vi "Write Operator.vi"(7 "Send any changes now? (F)":bool, 8 "error in (no error)":errorcluster, 10 "Operator":string caption="DUT Serial", 11 "Fiber Auto Collimation state data in":refnum<class "Fiber Auto Collimation state data.lvclass">) -> (0 "error out":errorcluster, 3 "Fiber Auto Collimation state data out":refnum<class "Fiber Auto Collimation state data.lvclass">)   [LabVIEW 2018, in "Fiber Auto Collimation state data.lvclass"]
doc: "Serial number of the Device Under Test on the station at the moment."
uses:
  Fiber Auto Collimation state data.lvclass
  Fiber Auto Collimation state data.lvclass/Fiber Auto Collimation state data.ctl
  Tracked state data.ctl
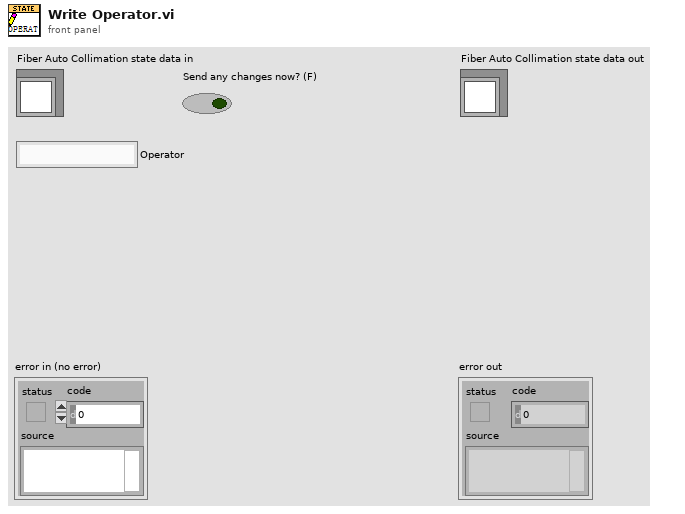
[diagram p1: front panel]
types:
  T1 = typedef "Fiber Auto Collimation state data.lvclass/Tracked state data.ctl" = enum16{"No update", "Permission level", "Username", "Test running", "DUT Serial", "Test status", "MOM Lot", "Loaded test recipe", "Model case running", "Station status", "BV data", "Defect Identify data", "Axis Position data", "Fiber Ass PN", "Operator", "RunTime", "VBAI", "Steps Cycle Time"}
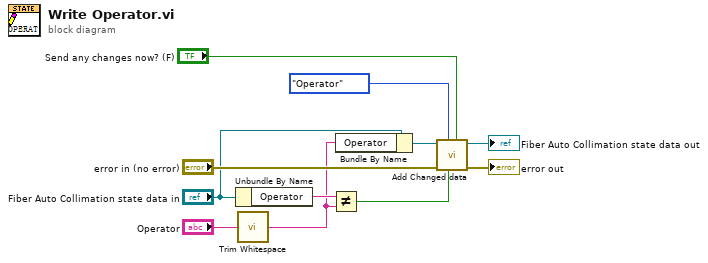
[diagram p0: block diagram]
diagram:
  n1 = Unbundle By Name("Fiber Auto Collimation state data in") -> ("Operator"=w3:string)
  n2 = call <vilib>:"Trim Whitespace.vi"("string"="Operator") -> ("trimmed string"=w2:string)  [unwired: 1 in]
  n3 = Not Equal?(x=w3, y=w2) -> (x != y?=w4:bool)
  n4 = Bundle By Name(cluster="Fiber Auto Collimation state data in", "Operator"=w2) -> (w7:refnum<class "Fiber Auto Collimation state data.lvclass">)
  n5 = call "Add Changed data.vi"("Send any changes now? (F)"="Send any changes now? (F)", "Data changed?"=w4, "Data type"=Tracked_state_data."Operator", "error in (no error)"="error in (no error)", "Fiber Auto Collimation state data in"=w7) -> ("error out"=→"error out":errorcluster, "Fiber Auto Collimation state data out"=→"Fiber Auto Collimation state data out":refnum<class "Fiber Auto Collimation state data.lvclass">)  [unwired: 5 in]
